vi "calc_multiManipJumpWaveform_v0.02.vi"(0 "New input cluster":T2={"Start Position (N)"=enum."Jumper Position C", "Duration (s)"=20.0, "Delay (s)"=2.0, "Valve 1 Position"=2, "Valve 2 Position"=2, "Replicates"=5.0, "Vholding (mV)"=-60.0, "Valve 3 Position"=2, "valve 1 used now?"=TRUE, "valve 2 used now?"=FALSE, "valve 3 used now? "=FALSE, "Jump Position Array"=[enum."Jumper Position B", enum."Jumper Position A", enum."Jumper Position B", enum."Jumper Position C"], "Position Dwell Time (s)"=[2.0, 4.0, 4.0, 4.0], "protocol Preview"=[]} {"Position Dwell Time (s)" min=0.0 step=0.1}, 1 "Clear Waveform?":bool, 5 "Old input cluster":T2={"Start Position (N)"=enum."Jumper Position C", "Duration (s)"=20.0, "Delay (s)"=2.0, "Valve 1 Position"=2, "Valve 2 Position"=2, "Replicates"=5.0, "Vholding (mV)"=-60.0, "Valve 3 Position"=2, "valve 1 used now?"=TRUE, "valve 2 used now?"=FALSE, "valve 3 used now? "=FALSE, "Jump Position Array"=[enum."Jumper Position B", enum."Jumper Position A", enum."Jumper Position B", enum."Jumper Position C"], "Position Dwell Time (s)"=[2.0, 4.0, 4.0, 4.0], "protocol Preview"=[]} {"Position Dwell Time (s)" min=0.0 step=0.1}, 7 "Numeric":i32=10000, 11 "error in":errorcluster) -> (4 "output cluster":T2={"Start Position (N)"=enum."Jumper Position C", "Duration (s)"=20.0, "Delay (s)"=2.0, "Valve 1 Position"=2, "Valve 2 Position"=2, "Replicates"=5.0, "Vholding (mV)"=-60.0, "Valve 3 Position"=2, "valve 1 used now?"=TRUE, "valve 2 used now?"=FALSE, "valve 3 used now? "=FALSE, "Jump Position Array"=[enum."Jumper Position B", enum."Jumper Position A", enum."Jumper Position B", enum."Jumper Position C"], "Position Dwell Time (s)"=[2.0, 4.0, 4.0, 4.0], "protocol Preview"=[]} {"Position Dwell Time (s)" min=0.0 step=0.1}, 15 "error out":errorcluster)   [LabVIEW 2019]
uses:
  <vilib>/measure/NI_MABase.lvlib
panel:
  out "PositionClusterArray":T1(array[cluster])
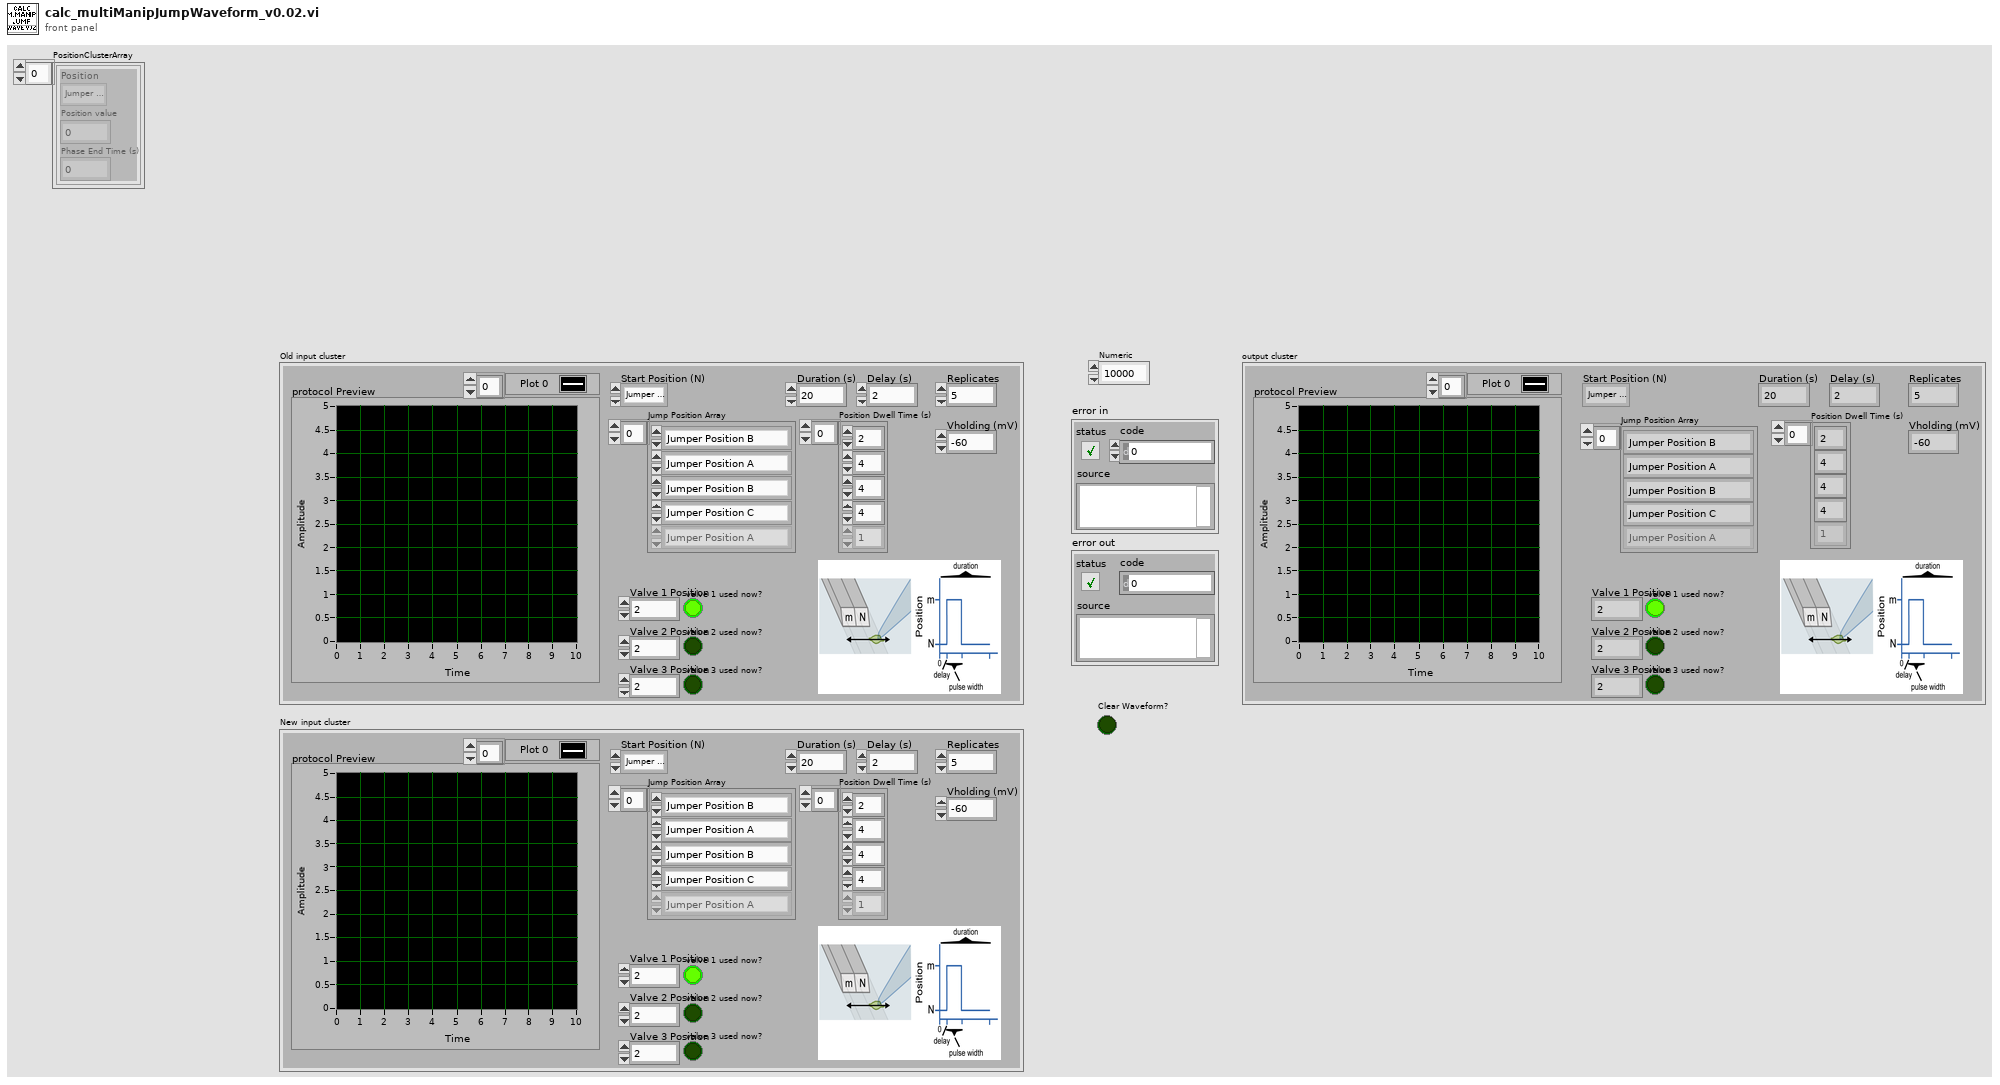
[diagram p1: front panel]
types:
  T1 = cluster{"Position":enum16{"Jumper Safe Position", "Experiment Safe Position", "Jumper Position A", "Jumper Position B", "Jumper Position C", "Jumper Position o-A", "Jumper Position A-o", "Jumper Position A-B", "Jumper Position B-A", "Jumper Position B-C", "Jumper Position C-B", "Jumper Position C-o", "Jumper Position o-C"}, "Position value":i32, "Phase End Time (s)":dbl}[]
  T2 = cluster{"Start Position (N)":enum16{"Jumper Safe Position", "Experiment Safe Position", "Jumper Position A", "Jumper Position B", "Jumper Position C", "Jumper Position o-A", "Jumper Position A-o", "Jumper Position A-B", "Jumper Position B-A", "Jumper Position B-C", "Jumper Position C-B", "Jumper Position C-o", "Jumper Position o-C"}, "Duration (s)":dbl, "Delay (s)":dbl, "Valve 1 Position":i16, "Valve 2 Position":i16, "Replicates":dbl, "Vholding (mV)":dbl, "Valve 3 Position":i16, "valve 1 used now?":bool, "valve 2 used now?":bool, "valve 3 used now? ":bool, "Jump Position Array":enum16{"Jumper Safe Position", "Experiment Safe Position", "Jumper Position A", "Jumper Position B", "Jumper Position C", "Jumper Position o-A", "Jumper Position A-o", "Jumper Position A-B", "Jumper Position B-A", "Jumper Position B-C", "Jumper Position C-B", "Jumper Position C-o", "Jumper Position o-C"}[], "Position Dwell Time (s)":dbl[], "protocol Preview":waveform(dbl)[]}
  T3 = cluster{"Position":enum16{"Jumper Safe Position", "Experiment Safe Position", "Jumper Position A", "Jumper Position B", "Jumper Position C", "Jumper Position o-A", "Jumper Position A-o", "Jumper Position A-B", "Jumper Position B-A", "Jumper Position B-C", "Jumper Position C-B", "Jumper Position C-o", "Jumper Position o-C"}, "Position value":i32, "Phase End Time (s)":dbl}
  T4 = enum16{"Jumper Safe Position", "Experiment Safe Position", "Jumper Position A", "Jumper Position B", "Jumper Position C", "Jumper Position o-A", "Jumper Position A-o", "Jumper Position A-B", "Jumper Position B-A", "Jumper Position B-C", "Jumper Position C-B", "Jumper Position C-o", "Jumper Position o-C"}
  T5 = enum16{"Jumper Safe Position", "Experiment Safe Position", "Jumper Position A", "Jumper Position B", "Jumper Position C", "Jumper Position o-A", "Jumper Position A-o", "Jumper Position A-B", "Jumper Position B-A", "Jumper Position B-C", "Jumper Position C-B", "Jumper Position C-o", "Jumper Position o-C"}[]
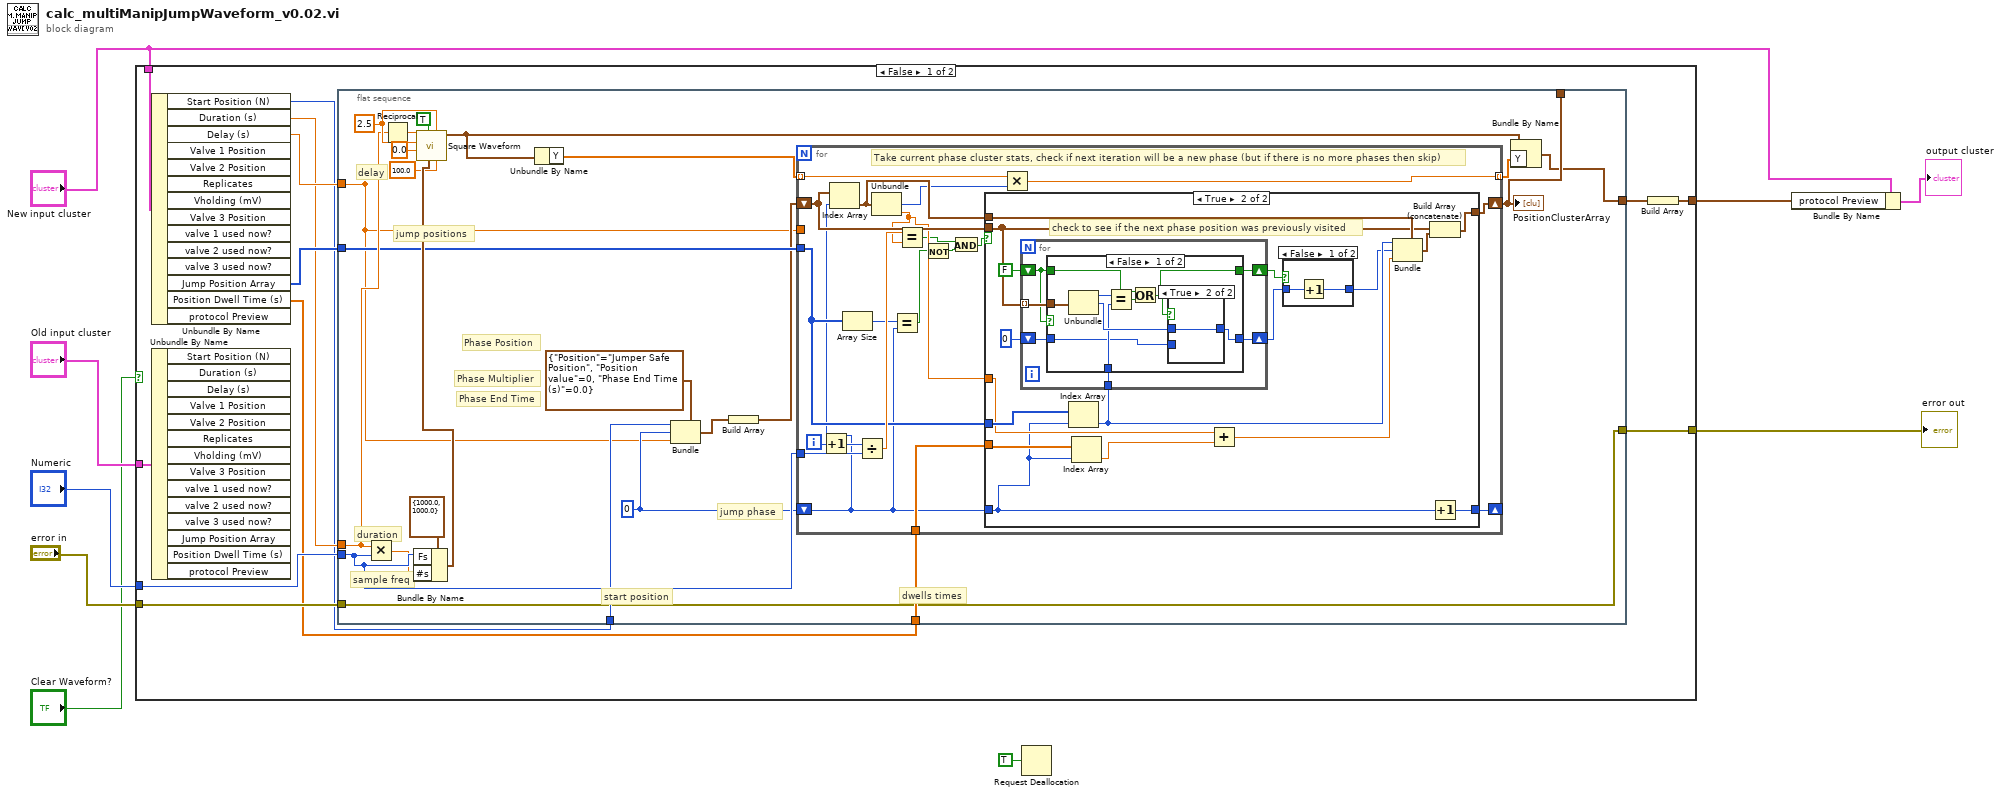
[diagram p0: block diagram]
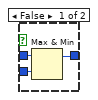
[diagram p4: hidden frame]
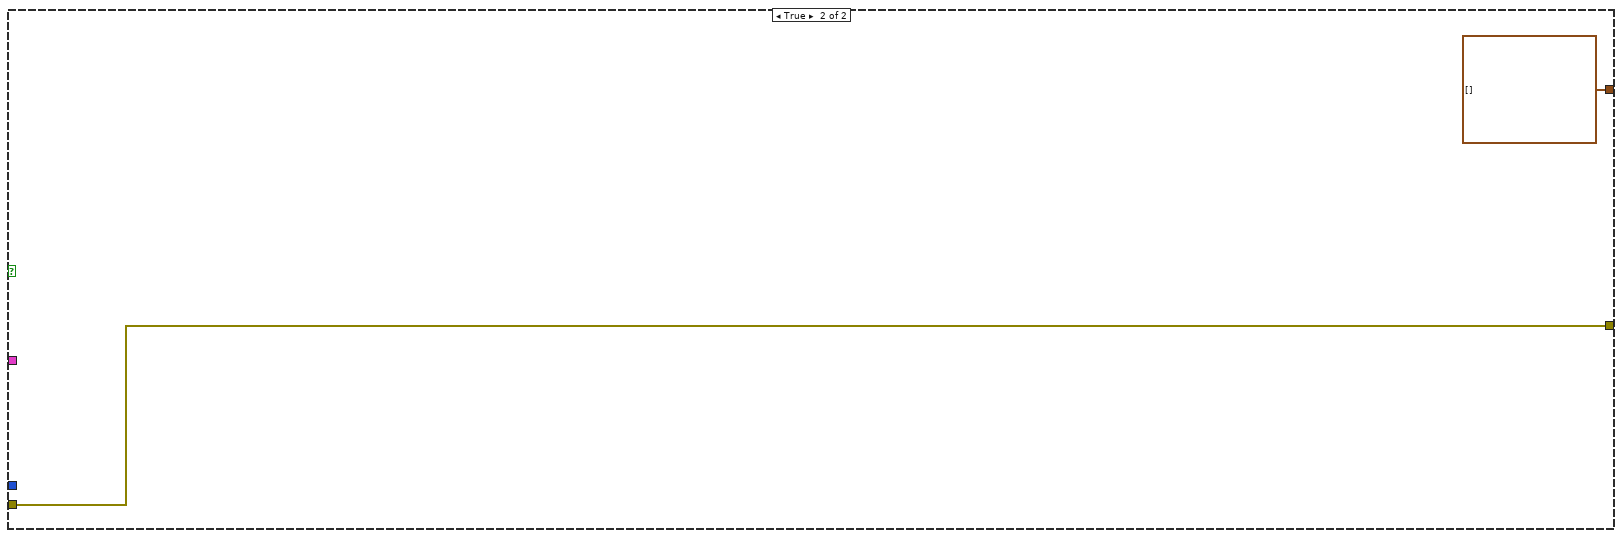
[diagram p6: hidden frame]
diagram:
  n1 = case shown="False" "Clear Waveform?" {
    tunnel: "New input cluster" -> [w21 _]
    tunnel: "Old input cluster" -> [w20 _]
    tunnel: [w19 waveform(dbl)[] []] -> w6
    tunnel: "error in" -> [w15 w109]
    tunnel: "Numeric" -> [w14 _]
    tunnel: [w10 w109] -> w3
    frame False {
      n2 = Unbundle By Name(w21) -> ("Start Position (N)"=w13:T4, "Duration (s)"=w16:dbl, "Delay (s)"=w17:dbl, "Jump Position Array"=w18:T5, "Position Dwell Time (s)"=w12:dbl[])  [unwired: 9 out]
      n3 = Unbundle By Name(w20) -> ()  [unwired: 14 out]
      n4 = flat-sequence {
        tunnel: [w24] -> _
        tunnel: w16 -> [w40]
        tunnel: w14 -> [w34]
        tunnel: w15 -> [w22]
        tunnel: w18 -> [w32]
        tunnel: w13 -> [w31]
        tunnel: w12 -> [w27]
        tunnel: [w25] -> _
        tunnel: w17 -> [w24]
        tunnel: [w23] -> w11
        tunnel: [w22] -> w10
        frame #0 {
          w30 = 0
          w45 = 2.5 ("Amplitude")
          # "dwells times"
          # "start position"
          # "duration"
          # "sample freq"
          # "jump positions"
          # "delay"
          # "Phase End Time"
          # "Phase Multiplier"
          # "Phase Position"
          # "jump phase"
          n5 = Multiply(x=w40, y=w34) -> (x*y=w33:dbl)
          n6 = Reciprocal(x=w40) -> (1/x=w41:dbl)
          n7 = Bundle By Name(cluster=cluster{"Fs":dbl, "#s":dbl} {"Fs"=1000.0, "#s"=1000.0} ("sampling info"), "Fs"=w34, "#s"=w33) -> (w42:cluster{"Fs":dbl, "#s":dbl})
          n8 = call <vilib>:"Square Waveform.vi"("duty cycle (%)"=100.0, "offset"=w45, "sampling info"=w42, "reset signal"=TRUE, "phase"=0.0, "amplitude"=w45, "frequency"=w41) -> ("signal out"=w37:waveform(dbl))  [unwired: 3 in, 1 out]
          n9 = Unbundle By Name(w37) -> ("Y"=w36:dbl[])
          n10 = Bundle(cluster=T3 {"Position"=enum."Jumper Safe Position", "Position value"=0, "Phase End Time (s)"=0.0} ("PositionsPhaseCluster"), "Position"=w31, "Position value"=w30, "Phase End Time (s)"=w24) -> (w29:T3)
          n11 = Build Array(w29) -> (w28:T1)
          n12 = for {
            tunnel: w36 -> [w65] mode=indexing
            tunnel: [w62] -> w35 mode=indexing
            tunnel: w34 -> [w63]
            tunnel: w24 -> [_]
            tunnel: w32 -> [w52]
            shift-right: [w61] -> _
            shift-left: w30 -> [w50]
            shift-right: [w57] -> w25
            shift-left: w28 -> [w58]
            tunnel: w27 -> [w53]
            i -> [w64]
            # "Take current phase cluster stats, check if next iteration will be a new phase (but if there is no more phases then skip)"
            n13 = Increment(x=w64) -> (x+1=w60:i32)
            n14 = Index Array(array=w58, index=w50) -> (element=w56:T3)
            n15 = Array Size(array=w52) -> (size(s)=w51:i32)
            n16 = Divide(x=w60, y=w63) -> (x/y=w59:dbl)
            n17 = Unbundle(w56) -> ("Position value"=w54:i32, "Phase End Time (s)"=w55:dbl)  [unwired: 1 out]
            n18 = Equal?(x=w51, y=w50) -> (x = y?=w47:bool)
            n19 = Equal?(x=w59, y=w55) -> (x = y?=w48:bool)
            n20 = Not(x=w47) -> (.not. x?=w46:bool)
            n21 = And(x=w48, y=w46) -> (x .and. y?=w49:bool)
            n22 = case shown="True" w49 {
              tunnel: w50 -> [w67 w68]
              tunnel: [w67 w84] -> w61
              tunnel: w58 -> [w66 w75]
              tunnel: [w66 w83] -> w57
              tunnel: w56 -> [_ w82]
              tunnel: w55 -> [_ w78]
              tunnel: w52 -> [_ w80]
              tunnel: w53 -> [_ w79]
              frame False {
              }
              frame True {
                # "check to see if the next phase position was previously visited"
                n23 = Index Array(array=w80, index=w68) -> (element=w74:T4)
                n24 = for {
                  tunnel: w75 -> [w93] mode=indexing
                  tunnel: w74 -> [w91]
                  shift-right: [w92] -> w70
                  shift-left: 0 -> [w90]
                  shift-right: [w89] -> w72
                  shift-left: FALSE ("x = y?") -> [w88]
                  n25 = case shown="False" w88 {
                    tunnel: w93 -> [w102 _]
                    tunnel: [w100 w107] -> w92
                    tunnel: w91 -> [w98 _]
                    tunnel: w90 -> [w97 w107]
                    tunnel: w88 -> [w95 w108]
                    tunnel: [w94 w108] -> w89
                    frame False {
                      n26 = Unbundle(w102) -> ("Position"=w99:T4, "Position value"=w101:i32)  [unwired: 1 out]
                      n27 = Equal?(x=w99, y=w98) -> (x = y?=w96:bool)
                      n28 = Or(x=w95, y=w96) -> (x .or. y?=w94:bool)
                      n29 = case shown="True" w94 {
                        tunnel: w101 -> [w104 w106]
                        tunnel: [w103 w106] -> w100
                        tunnel: w97 -> [w105 _]
                        frame False {
                          n30 = Max & Min(x=w104, y=w105) -> (max(x,y)=w103:i32)  [unwired: 1 out]
                        }
                        frame True {
                        }
                      }
                    }
                    frame True {
                    }
                  }
                }
                n31 = Index Array(array=w79, index=w68) -> (element=w76:dbl)
                n32 = Add(x=w78, y=w76) -> (x+y=w77:dbl)
                n33 = case shown="False" w72 {
                  tunnel: w70 -> [w86 w87]
                  tunnel: [w85 w87] -> w71
                  frame False {
                    n34 = Increment(x=w86) -> (x+1=w85:i32)
                  }
                  frame True {
                  }
                }
                n35 = Bundle(cluster=w82, "Position"=w74, "Position value"=w71, "Phase End Time (s)"=w77) -> (w81:T3)
                n36 = Build Array (concatenate)(w75, w81) -> (w83:T1)
                n37 = Increment(x=w68) -> (x+1=w84:i32)
              }
            }
            n38 = Multiply(x=w65, y=w54) -> (x*y=w62:dbl)
          }
          "PositionClusterArray" <- w25
          n39 = Bundle By Name(cluster=w37, "Y"=w35) -> (w23:waveform(dbl))
        }
      }
      n40 = Build Array(w11) -> (w19:waveform(dbl)[])
    }
    frame True {
    }
  }
  "error out" <- w3
  n41 = Request Deallocation(TRUE ("flag")) -> ()
  n42 = Bundle By Name(cluster="New input cluster", "protocol Preview"=w6) -> (→"output cluster":T2)
